vi "31_05_22.vi"() -> ()   [LabVIEW 2021]
uses:
  <vilib>/Utility/miscctls.llb/LVBoundsTypeDef.ctl
panel:
  out "XY Graph":cluster{dbl[], dbl[]}(graph)
  out "Waveform Graph 2":dbl[](graph)
  out "Waveform Graph":dbl[](graph)
  in  "Stop":bool
  out "2D Picture":picture
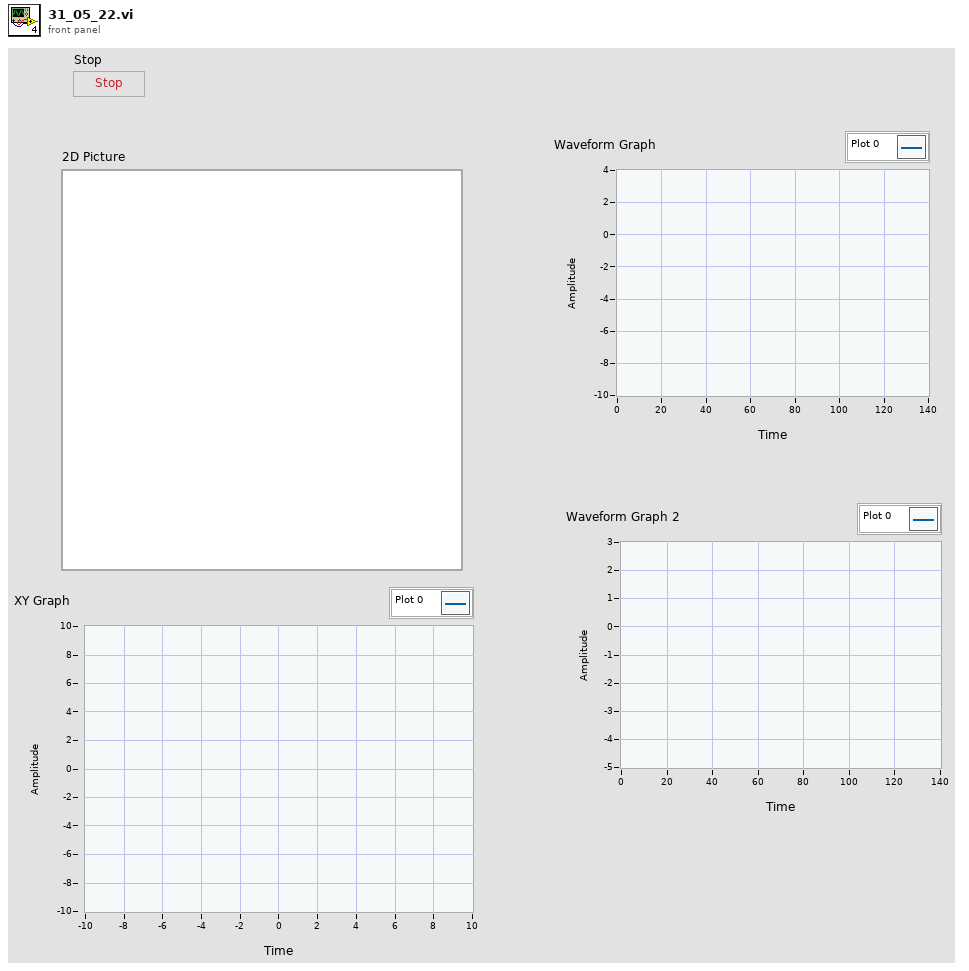
[diagram p1: front panel]
types:
  T1 = typedef "LVBoundsTypeDef.ctl" = cluster{"Width":u32, "Height":u32}
  T2 = typedef "LVMouseTypeDef.ctl" = cluster{"Mouse Position":cluster{"X":i32, "Y":i32}, "Mouse Modifiers":cluster{"Button Down":bool, "Shift Mod":bool, "Menu Mod":bool, "Option Mod":bool}}
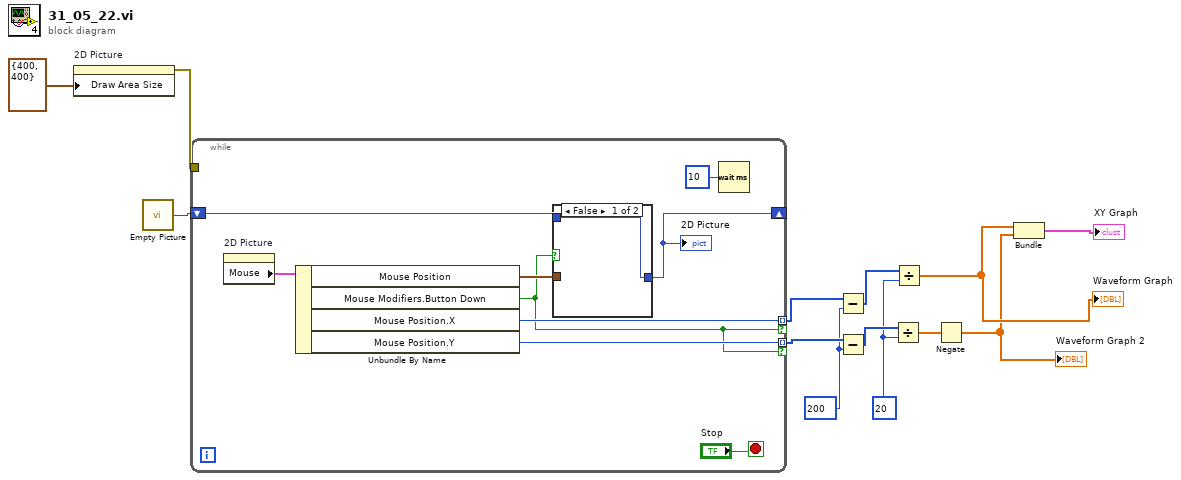
[diagram p0: block diagram]
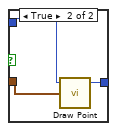
[diagram p2: hidden frame]
diagram:
  w4 = 20
  w7 = 200
  n1 = property on="2D Picture" class="Pict"("Draw Area Size"=T1 {"Width"=400, "Height"=400}) -> (error out=w11:errorcluster)  [unwired: 2 in, 1 out]
  n2 = call "Empty Picture"() -> ("empty picture"=w13:picture)
  n3 = while {
    shift-right: [w18] -> _
    shift-left: w13 -> [w17]
    tunnel: [w16] -> w9 mode=indexing if=w14
    tunnel: [w15] -> w8 mode=indexing if=w14
    tunnel: w11 -> [_]
    stop <- "Stop" stop-if-true
    n4 = property on="2D Picture" class="Pict"() -> ("Mouse"=w20:T2)  [unwired: 2 in, 2 out]
    n5 = Unbundle By Name(w20) -> ("Mouse Position"=w19:cluster{"X":i32, "Y":i32}, "Mouse Modifiers.Button Down"=w14:bool, "Mouse Position.X"=w16:i32, "Mouse Position.Y"=w15:i32)
    n6 = case shown="False" w14 {
      tunnel: w19 -> [_ w26]
      tunnel: [w23 w25] -> w18
      tunnel: w17 -> [w23 w24]
      frame False {
      }
      frame True {
        n7 = call <vilib>:"Draw Point.vi"("picture"=w24, "point(x,y)"=w26) -> ("new picture"=w25:picture)  [unwired: 7 in]
      }
    }
    "2D Picture" <- w18
    n8 = Wait (ms)(milliseconds to wait=u32 10) -> ()  [unwired: 1 out]
  }
  n9 = Subtract(x=w9, y=w7) -> (x-y=w6:i32[])
  n10 = Subtract(x=w8, y=w7) -> (x-y=w5:i32[])
  n11 = Divide(x=w5, y=w4) -> (x/y=w2:dbl[])
  n12 = Divide(x=w6, y=w4) -> (x/y=w3:dbl[])
  "Waveform Graph" <- w3
  n13 = Negate(x=w2) -> (-x=w1:dbl[])
  "Waveform Graph 2" <- w1
  n14 = Bundle(w3, w1) -> (→"XY Graph":cluster{dbl[], dbl[]})  [unwired: 1 in]
